vi "Dialog - Configure Packet Header.vi"(8 "error in (no error)":errorcluster, 9 "Header Elements In":bool[](array[boolean]), 11 "Packet Ref in":T1 format="%.0x") -> (0 "error out":errorcluster, 1 "Header Elements Out":bool[](array[boolean]), 3 "Packet Ref out":T1 format="%.0x")   [LabVIEW 2019, in "UDP-Custom-Device System Explorer.lvlib"]
uses:
  UDP-Custom-Device System Explorer.lvlib
  <vilib>/NI VeriStand/Custom Device API/Custom Device Item Ref.ctl
  <vilib>/NI VeriStand/Custom Device API/Custom Device API.lvlib
panel:
  in  "Source Node Name":bool
  in  "System Definition Version":bool
  in  "Protocol Revision":bool
  in  "Packet Size":bool=TRUE
  in  "TimeStamp":bool
  out "Data Header":string="Data"
  out "Num Bits Header":string="Num Bits"
  out "Data":string
  out "Num Bits":string
  in  "Cancel":bool
  in  "OK":bool
  in  "Packet Sequence":bool
  in  "Packet ID":bool
  in  "Num of Chans":bool
  # "Select Packet Header Information"
  # "Sample Packet Header"
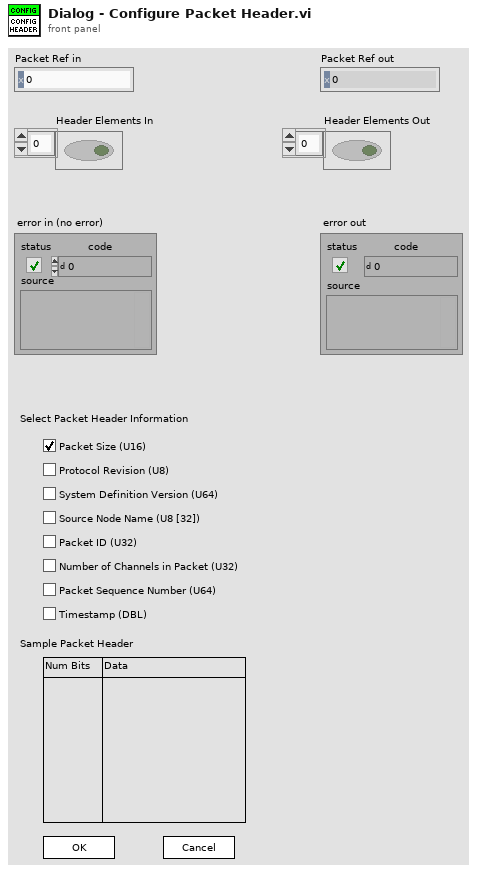
[diagram p1: front panel]
types:
  T1 = typedef "Custom Device API.lvlib/Custom Device Item Ref.ctl" = u64
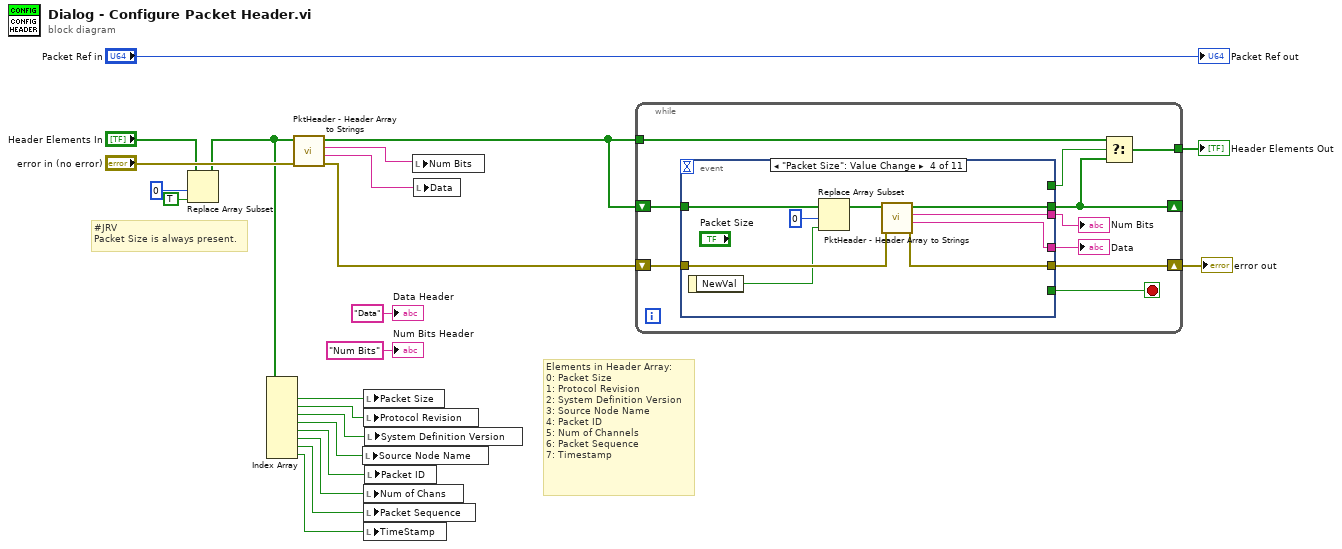
[diagram p0: block diagram]
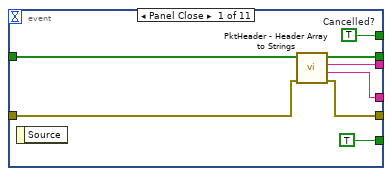
[diagram p2: hidden frame]
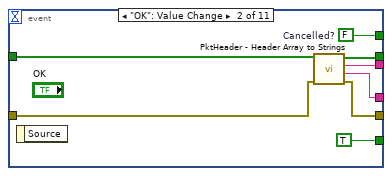
[diagram p3: hidden frame]
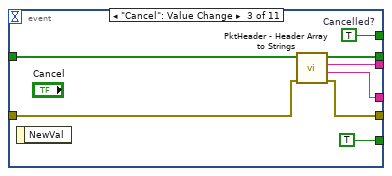
[diagram p4: hidden frame]
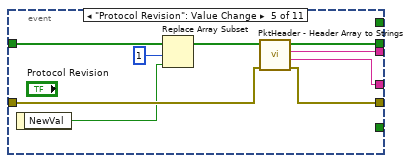
[diagram p5: hidden frame]
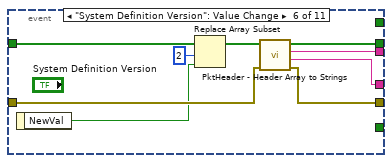
[diagram p6: hidden frame]
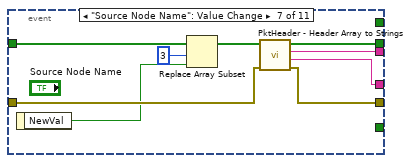
[diagram p7: hidden frame]
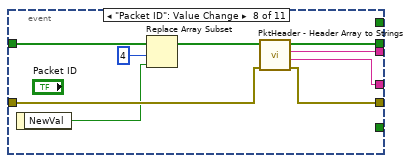
[diagram p8: hidden frame]
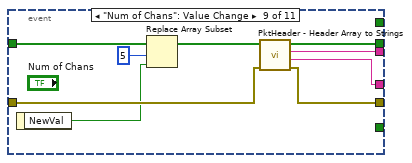
[diagram p9: hidden frame]
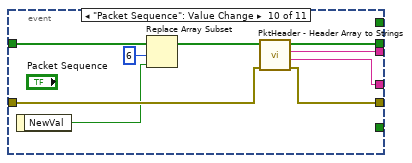
[diagram p10: hidden frame]
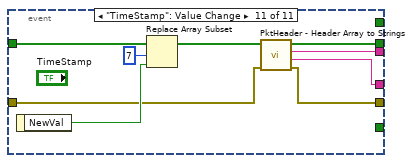
[diagram p11: hidden frame]
diagram:
  # "#JRV\nPacket Size is always present."
  # "Elements in Header Array:\n0: Packet Size\n1: Protocol Revision\n2: System Definition Version\n3: Source Node Name\n4: Packet ID\n5: Num of Channels\n6: Packet Sequence\n7: Timestamp"
  n1 = Replace Array Subset(array="Header Elements In", new element=TRUE ("new element/subarray"), index=0) -> (w2:bool[])
  n2 = Index Array(array=w2) -> (element #1=w12:bool, element #2=w11:bool, element #3=w10:bool, element #4=w9:bool, element #5=w8:bool, element #6=w7:bool, element #7=w6:bool, element #8=w5:bool)  [unwired: 8 in]
  n3 = call "PktHeader - Header Array to Strings.vi"("error in (no error)"="error in (no error)", "Header Array In"=w2) -> ("error out"=w13:errorcluster, "Data Name String"=w14:string, "Num Bits String"=w15:string, "Header Array Out"=w16:bool[])  [unwired: 6 in]
  n4 = local write "Source Node Name"(w9) -> ()
  n5 = local write "Packet Size"(w12) -> ()
  n6 = local write "Protocol Revision"(w11) -> ()
  n7 = local write "Num of Chans"(w7) -> ()
  n8 = local write "Packet Sequence"(w6) -> ()
  n9 = local write "TimeStamp"(w5) -> ()
  n10 = local write "System Definition Version"(w10) -> ()
  n11 = local write "Packet ID"(w8) -> ()
  n12 = local write "Num Bits"(w15) -> ()
  n13 = local write "Data"(w14) -> ()
  n14 = while {
    tunnel: w16 -> [w30]
    shift-right: [w27] -> _
    shift-left: w16 -> [w32]
    tunnel: [w29] -> w22
    shift-right: [w25] -> w18
    shift-left: w13 -> [w26]
    stop <- w31 stop-if-true
    n15 = event shown="[3] \"Packet Size\": Value Change" {
      selector: _ -> [_ _ _ _ _ _ _ _ _ _ _]
      dyn-events: _ -> [_ _ _ _ _ _ _ _ _ _ _]
      timeout: _ -> [_ _ _ _ _ _ _ _ _ _ _]
      tunnel: w32 -> [w38 w46 w54 w65 w74 w83 w92 w101 w110 w119 w128]
      tunnel: [w37 w45 w53 w62 w71 w80 w89 w98 w107 w116 w122] -> w27
      tunnel: [w40 w48 w56 _ _ _ _ _ _ _ _] -> w28
      tunnel: [TRUE TRUE TRUE _ _ _ _ _ _ _ _] -> w31
      tunnel: w26 -> [w33 w41 w49 w61 w70 w79 w88 w97 w106 w115 w124]
      tunnel: [w35 w43 w51 w60 w69 w78 w87 w96 w105 w114 w123] -> w25
      tunnel: [w36 w44 w52 w59 w68 w77 w86 w95 w104 w113 w121] -> w24
      tunnel: [w34 w42 w50 w58 w67 w76 w85 w94 w103 w112 w120] -> w23
      event Panel Close {
        w40 = TRUE  # Cancelled?
        n16 = event-data() -> ()  [unwired: 1 in, 1 out]
        n17 = call "PktHeader - Header Array to Strings.vi"("error in (no error)"=w33, "Header Array In"=w38) -> ("error out"=w35:errorcluster, "Data Name String"=w34:string, "Num Bits String"=w36:string, "Header Array Out"=w37:bool[])  [unwired: 6 in]
      }
      event "OK": Value Change {
        w48 = FALSE  # Cancelled?
        n18 = event-data() -> ()  [unwired: 1 in, 1 out]
        n19 = call "PktHeader - Header Array to Strings.vi"("error in (no error)"=w41, "Header Array In"=w46) -> ("error out"=w43:errorcluster, "Data Name String"=w42:string, "Num Bits String"=w44:string, "Header Array Out"=w45:bool[])  [unwired: 6 in]
      }
      event "Cancel": Value Change {
        w56 = TRUE  # Cancelled?
        n20 = event-data() -> ()  [unwired: 1 in, 1 out]
        n21 = call "PktHeader - Header Array to Strings.vi"("error in (no error)"=w49, "Header Array In"=w54) -> ("error out"=w51:errorcluster, "Data Name String"=w50:string, "Num Bits String"=w52:string, "Header Array Out"=w53:bool[])  [unwired: 6 in]
      }
      event "Packet Size": Value Change {
        n22 = event-data() -> ("NewVal"=w57:bool)  [unwired: 1 in]
        n23 = Replace Array Subset(array=w65, new element=w57, index=0) -> (w63:bool[])
        n24 = call "PktHeader - Header Array to Strings.vi"("error in (no error)"=w61, "Header Array In"=w63) -> ("error out"=w60:errorcluster, "Data Name String"=w58:string, "Num Bits String"=w59:string, "Header Array Out"=w62:bool[])  [unwired: 6 in]
      }
      event "Protocol Revision": Value Change {
        n25 = event-data() -> ("NewVal"=w66:bool)  [unwired: 1 in]
        n26 = Replace Array Subset(array=w74, new element=w66, index=1) -> (w72:bool[])
        n27 = call "PktHeader - Header Array to Strings.vi"("error in (no error)"=w70, "Header Array In"=w72) -> ("error out"=w69:errorcluster, "Data Name String"=w67:string, "Num Bits String"=w68:string, "Header Array Out"=w71:bool[])  [unwired: 6 in]
      }
      event "System Definition Version": Value Change {
        n28 = event-data() -> ("NewVal"=w75:bool)  [unwired: 1 in]
        n29 = Replace Array Subset(array=w83, new element=w75, index=2) -> (w81:bool[])
        n30 = call "PktHeader - Header Array to Strings.vi"("error in (no error)"=w79, "Header Array In"=w81) -> ("error out"=w78:errorcluster, "Data Name String"=w76:string, "Num Bits String"=w77:string, "Header Array Out"=w80:bool[])  [unwired: 6 in]
      }
      event "Source Node Name": Value Change {
        n31 = event-data() -> ("NewVal"=w84:bool)  [unwired: 1 in]
        n32 = Replace Array Subset(array=w92, new element=w84, index=3) -> (w90:bool[])
        n33 = call "PktHeader - Header Array to Strings.vi"("error in (no error)"=w88, "Header Array In"=w90) -> ("error out"=w87:errorcluster, "Data Name String"=w85:string, "Num Bits String"=w86:string, "Header Array Out"=w89:bool[])  [unwired: 6 in]
      }
      event "Packet ID": Value Change {
        n34 = event-data() -> ("NewVal"=w93:bool)  [unwired: 1 in]
        n35 = Replace Array Subset(array=w101, new element=w93, index=4) -> (w99:bool[])
        n36 = call "PktHeader - Header Array to Strings.vi"("error in (no error)"=w97, "Header Array In"=w99) -> ("error out"=w96:errorcluster, "Data Name String"=w94:string, "Num Bits String"=w95:string, "Header Array Out"=w98:bool[])  [unwired: 6 in]
      }
      event "Num of Chans": Value Change {
        n37 = event-data() -> ("NewVal"=w102:bool)  [unwired: 1 in]
        n38 = Replace Array Subset(array=w110, new element=w102, index=5) -> (w108:bool[])
        n39 = call "PktHeader - Header Array to Strings.vi"("error in (no error)"=w106, "Header Array In"=w108) -> ("error out"=w105:errorcluster, "Data Name String"=w103:string, "Num Bits String"=w104:string, "Header Array Out"=w107:bool[])  [unwired: 6 in]
      }
      event "Packet Sequence": Value Change {
        n40 = event-data() -> ("NewVal"=w111:bool)  [unwired: 1 in]
        n41 = Replace Array Subset(array=w119, new element=w111, index=6) -> (w117:bool[])
        n42 = call "PktHeader - Header Array to Strings.vi"("error in (no error)"=w115, "Header Array In"=w117) -> ("error out"=w114:errorcluster, "Data Name String"=w112:string, "Num Bits String"=w113:string, "Header Array Out"=w116:bool[])  [unwired: 6 in]
      }
      event "TimeStamp": Value Change {
        n43 = event-data() -> ("NewVal"=w126:bool)  [unwired: 1 in]
        n44 = Replace Array Subset(array=w128, new element=w126, index=7) -> (w125:bool[])
        n45 = call "PktHeader - Header Array to Strings.vi"("error in (no error)"=w124, "Header Array In"=w125) -> ("error out"=w123:errorcluster, "Data Name String"=w120:string, "Num Bits String"=w121:string, "Header Array Out"=w122:bool[])  [unwired: 6 in]
      }
    }
    "Num Bits" <- w24
    "Data" <- w23
    n46 = Select(t=w30, s=w28, f=w27) -> (s? t:f=w29:bool[])
  }
  "error out" <- w18
  "Header Elements Out" <- w22
  "Packet Ref out" <- "Packet Ref in"
  "Num Bits Header" <- "Num Bits" ("Num Bits Header")
  "Data Header" <- "Data" ("Data Header")
